vi "Log File Create.vi"(8 "error in":errorcluster, 10 "initial filename":string, 11 "base path":path) -> (0 "error out":errorcluster, 3 "refnum out":refnum<file>)   [LabVIEW 2019]
doc: "Create execution log file with the current date in the name preceded by <initial filename>."
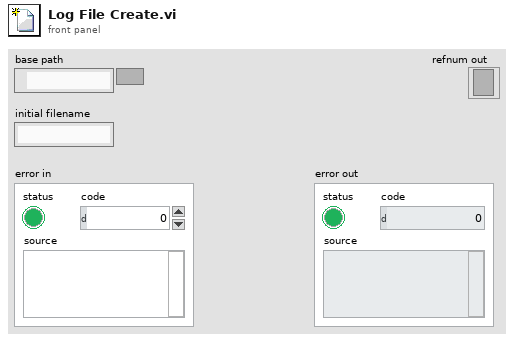
[diagram p1: front panel]
types:
  T1 = enum16{"open", "replace", "create", "open or create", "replace or create", "replace or create with confirmation"}
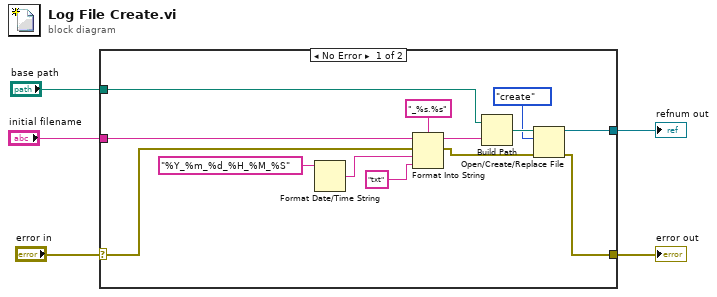
[diagram p0: block diagram]
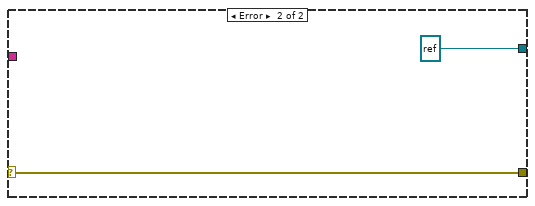
[diagram p2: hidden frame]
diagram:
  n1 = case shown="No Error" "error in" {
    selector: "error in" -> [w12 w20]
    tunnel: "base path" -> [w9 _]
    tunnel: "initial filename" -> [w8 _]
    tunnel: [w7 w20] -> w2
    tunnel: [w6 refnum<file> refnum ("refnum out")] -> w1
    frame No Error {
      n2 = Format Date/Time String(time format string (%c)="%Y_%m_%d_%H_%M_%S") -> (date/time string=w16:string)  [unwired: 2 in]
      n3 = Format Into String(format string="_%s.%s", initial string=w8, error in=w12, w16, "txt" ("input 2")) -> (resulting string=w15:string, error out=w11:errorcluster)
      n4 = Build Path(base path=w9, name or relative path=w15) -> (appended path=w14:path)
      n5 = Open/Create/Replace File(file path (use dialog)=w14, error in=w11, operation (0:open)=T1."create") -> (refnum out=w6:refnum<file>, error out=w7:errorcluster)  [unwired: 3 in, 1 out]
    }
    frame Error {
    }
  }
  "error out" <- w2
  "refnum out" <- w1
